vi "unregGenReadUserEvent.vi"(8 "error in (no error)":errorcluster, 11 "tcpServerBase in":refnum<class "TcpServerBase.lvclass">) -> (0 "error out":errorcluster, 3 "tcpServerBase out":refnum<class "TcpServerBase.lvclass">)   [LabVIEW 2018, in "TcpServerBase.lvclass"]
doc: "Unregister the GenRead user event. \n\nNote: This will be used in TcpServerCmd only, because the user event reference id is the same for the children."
uses:
  TcpServerBase.lvclass
  TcpServerBase.lvclass/TcpServerBase.ctl
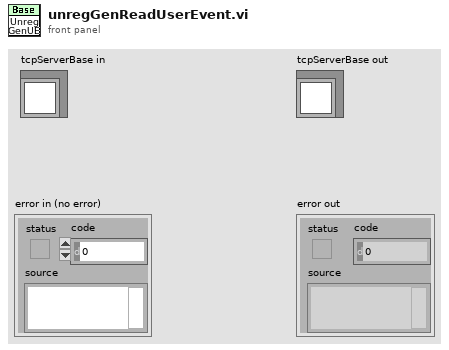
[diagram p1: front panel]
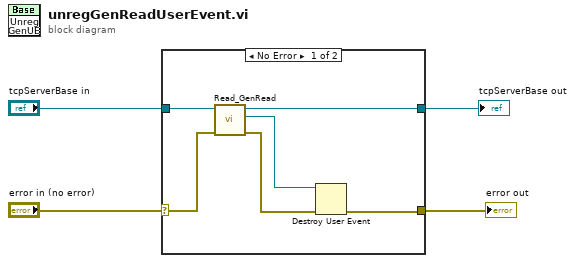
[diagram p0: block diagram]
diagram:
  n1 = case shown="No Error" "error in (no error)" {
    selector: "error in (no error)" -> [w10 w12]
    tunnel: [w9 w12] -> w3
    tunnel: [w6 w11] -> w1
    tunnel: "tcpServerBase in" -> [w7 w11]
    frame No Error {
      n2 = call "Read_GenRead.vi"("error in (no error)"=w10, "TcpServerBase in"=w7) -> ("error out"=w8:errorcluster, "GenRead"=w5:refnum<user-event>, "TcpServerBase out"=w6:refnum<class "TcpServerBase.lvclass">)  [unwired: 7 in]
      n3 = Destroy User Event(user event=w5, error in=w8) -> (error out=w9:errorcluster)
    }
    frame Error {
    }
  }
  "error out" <- w3
  "tcpServerBase out" <- w1
